vi "NF87xx.evt call Move 2 Pos.vi"(0 "i ref in":refnum<vi>, 1 "Instance":string="N/A", 2 "Position":i32, 3 "Immediately?":bool, 5 "error in (no error)":errorcluster, 6 "System":string="N/A") -> (14 "i ref out":refnum<vi>, 19 "error out":errorcluster)   [LabVIEW 2014, in "NF87XX.lvlib"]
doc: "This VI sets the \"SetAbsPosition\" case by a simple call. The instance has to be something else but N/A."
uses:
  NF87XX.lvlib
  CS_Core/CSSystem/CoreLib/CoreLib.short 2 byte array.vi
  CS_Core/CSSystem/CoreLib/CoreLib.int 2 byte array.vi
  CS_Core/CSSystem/CoreLib/CoreLib.string 2 byte array.vi
  CS_Core/BaseProcess/BaseProcess.lvlib
  CS_Core/CSSystem/CoreLib/CoreLib.lvlib
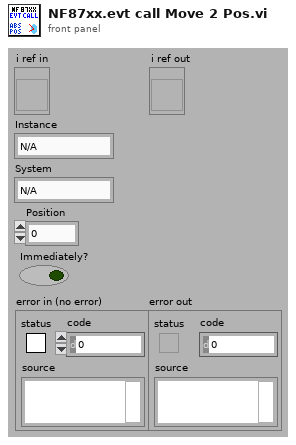
[diagram p1: front panel]
types:
  T1 = enum16{"simple", "synchronous", "asynchronous", "notification"}
  T2 = typedef "CoreDefs.rawDataType.ctl" = i8[]
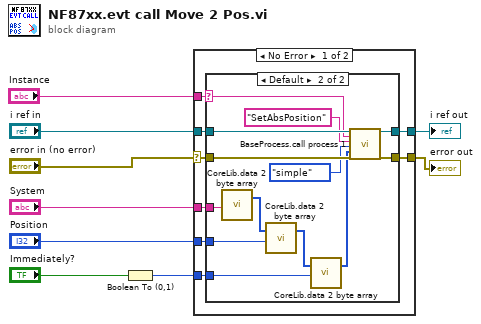
[diagram p0: block diagram]
diagram:
  n1 = Boolean To (0,1)(Boolean="Immediately?") -> (0, 1=w1:i16)
  n2 = case shown="No Error" "error in (no error)" {
    selector: "error in (no error)" -> [w11 w33]
    tunnel: [w17 w34] -> w9
    tunnel: [w16 w33] -> w8
    tunnel: "i ref in" -> [w15 w34]
    tunnel: "Position" -> [w14 _]
    tunnel: w1 -> [w13 _]
    tunnel: "Instance" -> [w12 _]
    tunnel: "System" -> [w10 _]
    frame No Error {
      n3 = case shown="Default" w12 {
        selector: w12 -> [_ w27]
        tunnel: [w19 w32] -> w17
        tunnel: [w18 w31] -> w16
        tunnel: w15 -> [w19 w30]
        tunnel: w11 -> [w18 w29]
        tunnel: w14 -> [_ w26]
        tunnel: w13 -> [_ w28]
        tunnel: w10 -> [_ w25]
        frame "N/A" {
        }
        frame Default {
          n4 = call-poly "CoreLib.data 2 byte array.vi"("string"=w25) -> ("byteArray out"=w21:T2)  [unwired: 18 in]
          n5 = call-poly "CoreLib.data 2 byte array.vi"("byteArray"=w21, "i32"=w26) -> ("byteArray out"=w22:T2)  [unwired: 17 in]
          n6 = call-poly "CoreLib.data 2 byte array.vi"("byteArray"=w22, "i16"=w28) -> ("byteArray out"=w20:T2)  [unwired: 17 in]
          n7 = call "BaseProcess.call process 1.vi"("i ref in"=w30, "Object"=w27, "Selector"="SetAbsPosition", "CallType"=T1."simple", "Data"=w20, "error in (no error)"=w29) -> ("i ref out"=w32:refnum<vi>, "error out"=w31:errorcluster)  [unwired: 11 in, 1 out]
        }
      }
    }
    frame Error {
    }
  }
  "error out" <- w8
  "i ref out" <- w9
